vi "Check-Manual-trigger.vi"(8 "error in":errorcluster, 10 "Acquis. params. ref.":refnum<data-value>, 11 "Manual trigger in":refnum<vi>) -> (0 "error IO":errorcluster)   [LabVIEW 2013, in "CameraVision.lvlib" / "CV-UI.lvclass"]
uses:
  CV-UI.lvclass
  Main/Acquisition/CV-Acquisition.lvclass
  Main/Acquisition/CV-Acquisition.lvclass/CV-Acquisition.ctl
  Main/Acquisition/Read Trigger mode.vi
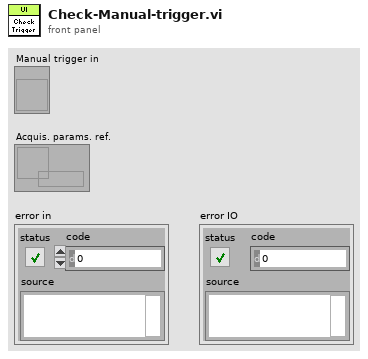
[diagram p1: front panel]
types:
  T1 = enum8{"Enabled", "Disabled", "Disabled and Grayed Out"}
  T2 = typedef "CameraVision.lvlib/Acquisition.lvclass/Trigger-modes.ctl" = enum16{"Camera timed (not sync.)", "Framegrabber timed (sync.)", "Software timed (sync.)", "External timing (sync.)", "Manual (sync.)", "Gated - camera (not sync.)", "Gated - grabber (sync.)", "Gated - software (sync.)", "Gated - external (sync.)"}
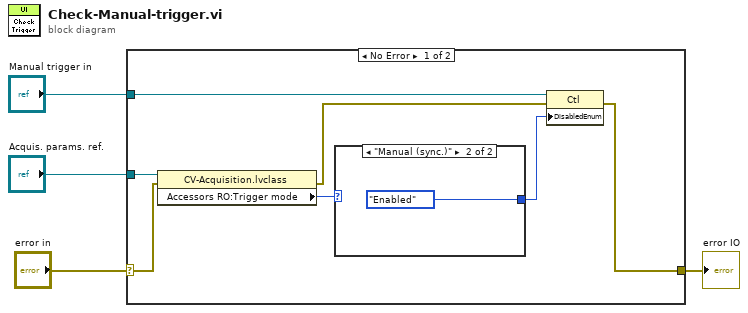
[diagram p0: block diagram]
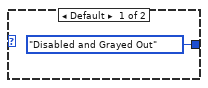
[diagram p2: hidden frame]
diagram:
  n1 = case shown="No Error" "error in" {
    selector: "error in" -> [w6 w14]
    tunnel: "Acquis. params. ref." -> [w11 _]
    tunnel: "Manual trigger in" -> [w9 _]
    tunnel: [w5 w14] -> w4
    frame No Error {
      n2 = property class="CV-Acquisition.lvclass"(reference=w11, error in=w6) -> (error out=w7:errorcluster, "Accessors RO:Trigger mode"=w10:T2)  [unwired: 1 out]
      n3 = case shown="\"Manual (sync.)\"" w10 {
        tunnel: [T1."Disabled and Grayed Out" ("Disabled") T1."Enabled" ("Disabled")] -> w8
        frame Default {
        }
        frame "Manual (sync.)" {
        }
      }
      n4 = property class="Ctl"(reference=w9, error in=w7, "DisabledEnum"=w8) -> (error out=w5:errorcluster)  [unwired: 1 out]
    }
    frame Error {
    }
  }
  "error IO" <- w4
